vi "Single FFT.vi"   [LabVIEW 2014]
uses:
  <vilib>/rvi/Analysis/measure/FFT/simModelSupport/niFPGA FFT Streaming Sim Properties.ctl
  <vilib>/rvi/Analysis/measure/FFT/simModelSupport/niFPGA FFT Sim Stream Group Properties.ctl
  <vilib>/rvi/Analysis/measure/FFT/simModelSupport/niFPGA FFT Sim Types.ctl
  <vilib>/rvi/Analysis/measure/FFT/simModelSupport/niFpgaFFTSimArithmeticProperties.ctl
  <vilib>/rvi/Analysis/measure/FFT/simModelSupport/niFpgaFFTSimDfxp.ctl
  <vilib>/fxp/LVFixedPointQuantizationPolicyTypeDef.ctl
  <vilib>/rvi/Analysis/measure/FFT/XNode/niFpgaFFTButterflyDelays.ctl
  <vilib>/rvi/interface/RandomDataEmulation/niFpgaRandomDataHandleErrors.vi
  <vilib>/rvi/Emulation/niFpgaEmulationIsFPGAContextNoSignature.vi
  <vilib>/rvi/Emulation/niFpgaSctlEmulationGetInTimedLoop.vi
  <vilib>/rvi/errors/niFpgaSetErrorForExecOnDevCompSimple.vi
  <vilib>/rvi/eio/common/nirviEmuReportErrorAndStop.vi
  <vilib>/rvi/DataTransferAndStorage/Container/Common/niFpgaContainerGetUniqueNameForEmu.vi
  <vilib>/rvi/FIFO/Fifo_Resource/nirvififoEmulationSetSize.vi
  <vilib>/rvi/FIFO/Fifo_Resource/nirviFifoEmulationQueueMgr.vi
  <instcachedir>/0/nirviFifoEmulationQueueMgr_E5CAEC123FF24DC58D834DCA3CDAA9B5.lvgen/nirviFifoEmulationQueueMgr_E5CAEC123FF24DC58D834DCA3CDAA9B5_010.vi
  <vilib>/rvi/FIFO/Fifo_Resource/nirvififoEmulationCreateLock.vi
  <vilib>/rvi/Emulation/niFpgaProcessEmulError.vi
  <vilib>/rvi/FIFO/Fifo_Resource/nirvififoEmulationObtainLock.vi
  <vilib>/rvi/FIFO/Fifo_Resource/nirvififoEmulationReleaseLock.vi
  <vilib>/rvi/occurrence/nirviWaitOnOccurrenceBase.vi
  <vilib>/rvi/errors/nirviReportUnexpectedCaseInternalError.vi
  <vilib>/rvi/errors/nirviReportUnexpectedCaseInternalError (U32).vi
  <vilib>/rvi/Analysis/measure/FFT/simModelSupport/niFpgaFFTSimModelStreamingCore.vi
  <vilib>/rvi/DataTransferAndStorage/Container/XNode/niFpgaContainer.xnode
  <vilib>/rvi/interface/RandomDataEmulation/nirviRandomDataFpgaReadWriteTemplate.vi
  <vilib>/rvi/FIFO/Fifo_Resource/nirvififoEmulationRead.vi
  <vilib>/rvi/Analysis/measure/FFT/XNode/niFpgaFFT.xnode
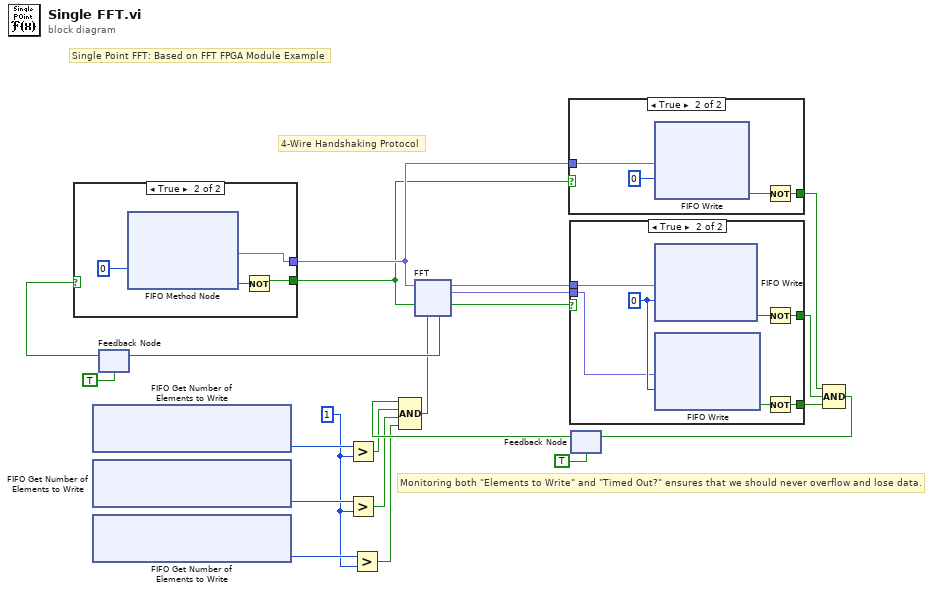
[diagram p0: block diagram]
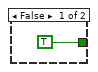
[diagram p2: hidden frame]
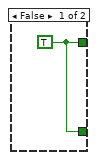
[diagram p3: hidden frame]
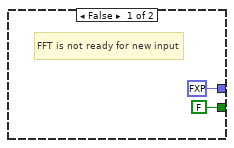
[diagram p4: hidden frame]
diagram:
  w8 = u32 1 ("y")
  # "Single Point FFT: Based on FFT FPGA Module Example"
  # "Monitoring both \"Elements to Write\" and \"Timed Out?\" ensures that we should never overflow and lose data."
  # "4-Wire Handshaking Protocol"
  n1 = xnode ("FIFO Get Number of Elements to Write")() -> ("Number of Elements to Write"=w11:u32)  [unwired: 1 in, 1 out]
  n2 = xnode ("FIFO Get Number of Elements to Write")() -> ("Number of Elements to Write"=w10:u32)  [unwired: 1 in, 1 out]
  n3 = xnode ("FIFO Get Number of Elements to Write")() -> ("Number of Elements to Write"=w9:u32)  [unwired: 1 in, 1 out]
  n4 = feedback #1(TRUE ("ready for input")) -> (w22:bool)
  n5 = case shown="True" w22 {
    tunnel: [FALSE w26] -> w19
    tunnel: [fxp<+/-,12,5> 0.0 ("Element") w25] -> w21
    frame False {
      # "FFT is not ready for new input"
    }
    frame True {
      n6 = xnode ("FIFO Method Node")("Timeout"=0) -> ("Element"=w25:fxp<+/-,12,12>, "Timed Out?"=w28:bool)  [unwired: 1 in, 1 out]
      n7 = Not(x=w28) -> (.not. x?=w26:bool)
    }
  }
  n8 = Greater?(x=w11, y=w8) -> (0:w5:bool)
  n9 = Greater?(x=w10, y=w8) -> (0:w4:bool)
  n10 = Greater?(x=w9, y=w8) -> (0:w3:bool)
  n11 = case shown="True" w19 {
    tunnel: w21 -> [_ w30]
    tunnel: [TRUE ("Timed Out?") w31] -> w15
    frame False {
    }
    frame True {
      n12 = xnode ("FIFO Write")("Element"=w30, "Timeout"=0) -> ("Timed Out?"=w32:bool)  [unwired: 1 in, 1 out]
      n13 = Not(x=w32) -> (.not. x?=w31:bool)
    }
  }
  n14 = feedback #2(TRUE) -> (w6:bool)
  n15 = Compound Arithmetic op=AND(w6, w5, w4, w3) -> (w7:bool)
  n16 = xnode "FFT"("real data in"=w21, "input valid"=w19, "ready for output"=w7) -> ("ready for input"=w20:bool, "real data out"=w18:fxp<+/-,29,22>, "imaginary data out"=w17:fxp<+/-,29,22>, "output valid"=w16:bool)  [unwired: 2 in, 1 out]
  n17 = feedback-in #1(w20) -> ()
  n18 = case shown="True" w16 {
    tunnel: w18 -> [_ w36]
    tunnel: w17 -> [_ w35]
    tunnel: [w34 w38] -> w14
    tunnel: [w34 w37] -> w13
    frame False {
      w34 = TRUE ("Timed Out?")
    }
    frame True {
      w41 = 0 ("Timeout")
      n19 = xnode ("FIFO Write")("Element"=w36, "Timeout"=w41) -> ("Timed Out?"=w40:bool)  [unwired: 1 in, 1 out]
      n20 = xnode ("FIFO Write")("Element"=w35, "Timeout"=w41) -> ("Timed Out?"=w39:bool)  [unwired: 1 in, 1 out]
      n21 = Not(x=w40) -> (.not. x?=w38:bool)
      n22 = Not(x=w39) -> (.not. x?=w37:bool)
    }
  }
  n23 = Compound Arithmetic op=AND(w15, w14, w13) -> (w1:bool)
  n24 = feedback-in #2(w1) -> ()
